vi "simple_pwm.vi"() -> ()   [LabVIEW 2017]
uses:
  lib/libbuddy/bindings/labview/utility_vi/buddy.lvlib
panel:
  out "Function Error":bool
  out "Configuration Error":bool
  out "output cluster":T1
  in  "packet":T1
  out "CH5":bool
  out "CH4":bool
  out "CH3":bool
  out "CH2":bool
  out "CH1":bool=TRUE
  out "function return":i32
  out "configure return":i32
  in  "Stream Mode":bool
  in  "PWM Mode":i32(listbox)=1
  in  "runtime":T2
  in  "CH5":u32(slide) max=65535 step=1 scale=0.0..65535.0
  in  "CH4":u32(slide) max=65535 step=1 scale=0.0..65535.0
  in  "CH3":u32(slide) max=65535 step=1 scale=0.0..65535.0
  in  "CH2":u32(slide) max=65535 step=1 scale=0.0..65535.0
  in  "CH1":u32(slide) max=65535 step=1 scale=0.0..65535.0
  in  "PWM Resolution":i32(listbox)=1
  out "PWM Sample Time":dbl
  in  "PWM Timebase":i32(listbox)=2
  out "Iterations":i32
  in  "stop":bool
  out "timing":cluster{"period":u32, "averaging":u8}
  in  "PWM Sample Rate (Hz)":dbl=10.0
  out "fw_info out":T3
  in  "timing":cluster{"period":u32, "averaging":u8}={"period"=1000000, "averaging"=0}
  in  "general":T4={"function"=2, "mode"=1, "channel_mask"=255, "resolution"=1}
  out "str_serial":string
  out "str_mfr":string
  out "str_product":string
  out "str_index_1":string
  out "handle":u64 format="%x"
  # "CONFIGURATION"
  # "DEVICE INFO"
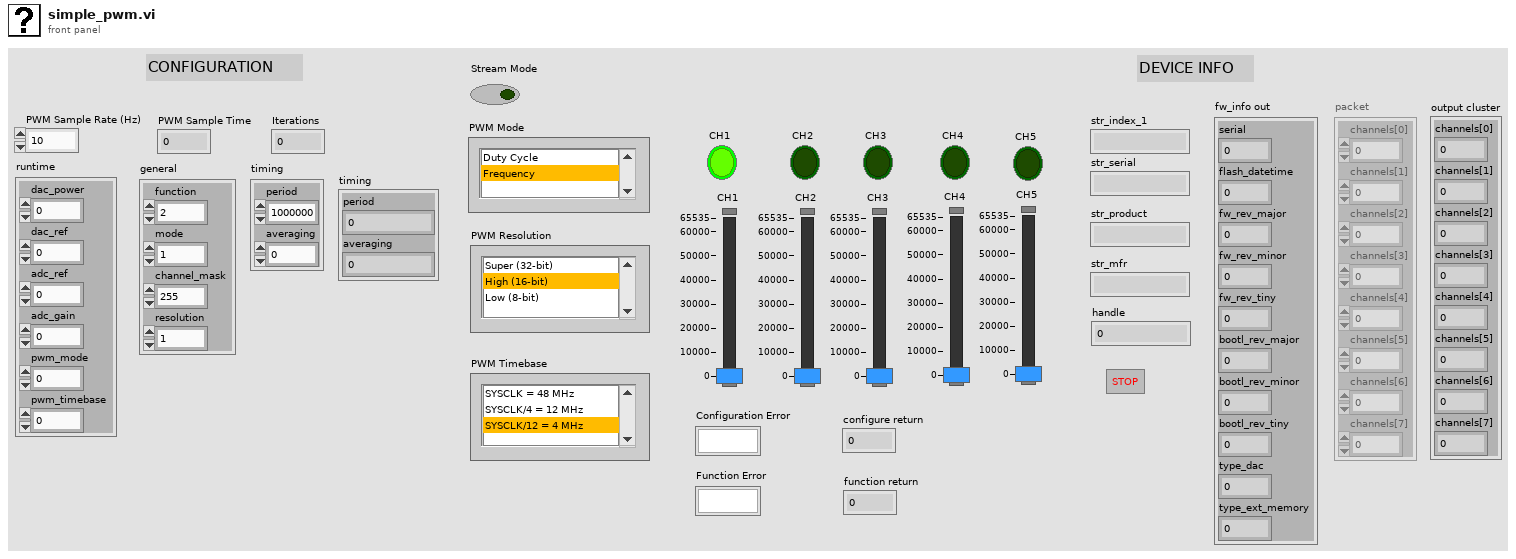
[diagram p1: front panel]
types:
  T1 = cluster{"channels[0]":u32, "channels[1]":u32, "channels[2]":u32, "channels[3]":u32, "channels[4]":u32, "channels[5]":u32, "channels[6]":u32, "channels[7]":u32}
  T2 = cluster{"dac_power":u8, "dac_ref":u8, "adc_ref":u8, "adc_gain":u8, "pwm_mode":u8, "pwm_timebase":u8}
  T3 = cluster{"serial":u32, "flash_datetime":u32, "fw_rev_major":u8, "fw_rev_minor":u8, "fw_rev_tiny":u8, "bootl_rev_major":u8, "bootl_rev_minor":u8, "bootl_rev_tiny":u8, "type_dac":u8, "type_ext_memory":u8}
  T4 = cluster{"function":u8, "mode":u8, "channel_mask":u8, "resolution":u8}
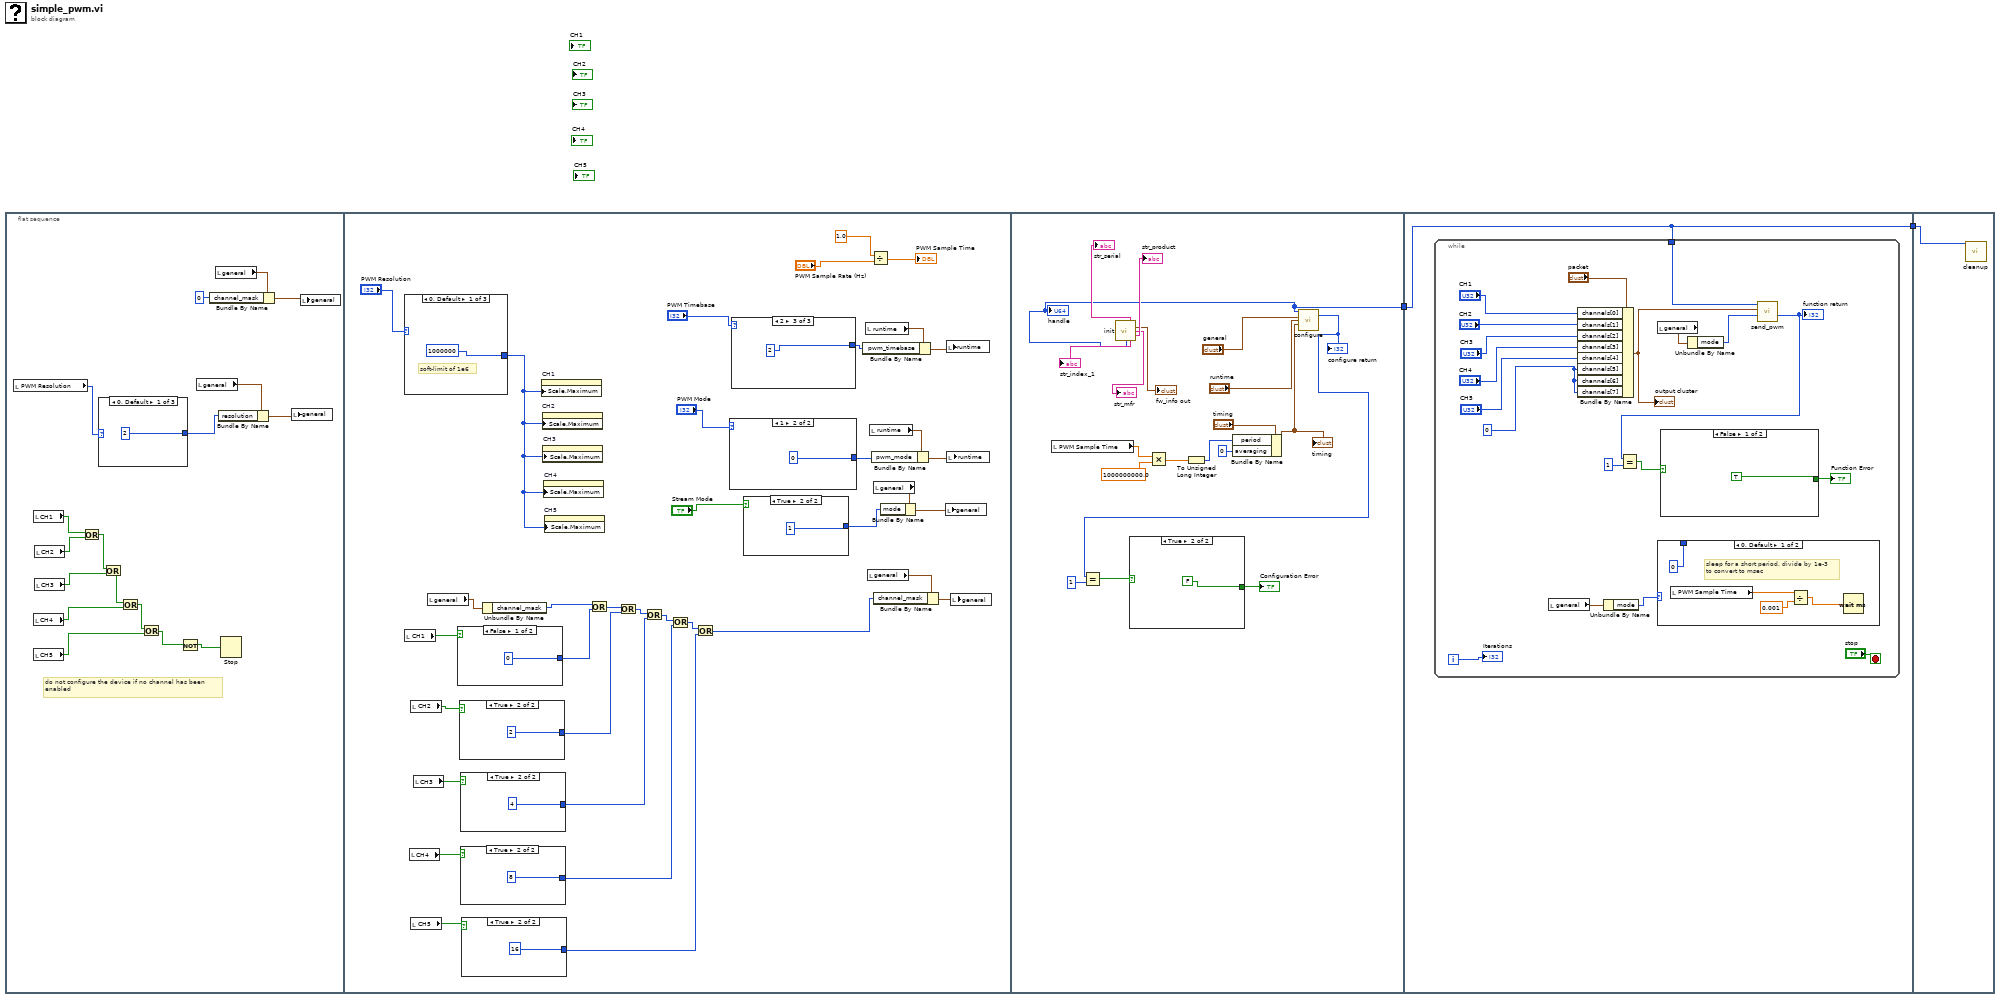
[diagram p0: block diagram]
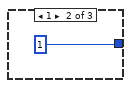
[diagram p2: hidden frame]
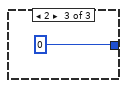
[diagram p3: hidden frame]
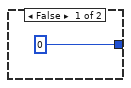
[diagram p4: hidden frame]
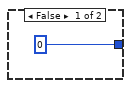
[diagram p5: hidden frame]
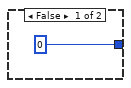
[diagram p6: hidden frame]
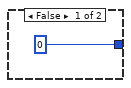
[diagram p7: hidden frame]
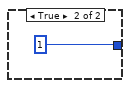
[diagram p8: hidden frame]
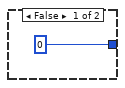
[diagram p9: hidden frame]
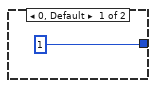
[diagram p10: hidden frame]
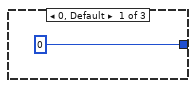
[diagram p11: hidden frame]
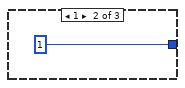
[diagram p12: hidden frame]
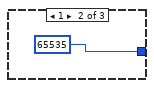
[diagram p13: hidden frame]
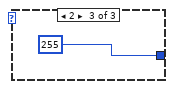
[diagram p14: hidden frame]
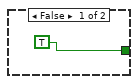
[diagram p15: hidden frame]
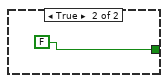
[diagram p16: hidden frame]
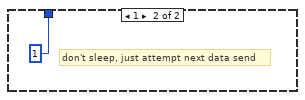
[diagram p17: hidden frame]
diagram:
  n1 = flat-sequence {
    tunnel: [w86] -> w1
    tunnel: [w100] -> w2
    tunnel: w1 -> [w100]
    tunnel: w2 -> [w127]
    frame #0 {
      # "do not configure the device if no channel has been\nenabled"
      n2 = local read "PWM Resolution"() -> (w14:i32)
      n3 = local read "CH1"() -> (w11:bool)
      n4 = local read "CH4"() -> (w7:bool)
      n5 = local read "CH5"() -> (w4:bool)
      n6 = local read "CH2"() -> (w10:bool)
      n7 = local read "CH3"() -> (w9:bool)
      n8 = Or(x=w11, y=w10) -> (x .or. y?=w8:bool)
      n9 = case shown="0, Default" w14 {
        tunnel: [u32 2 u32 1 u32 0] -> w13
        frame 0, Default {
        }
        frame 1 {
        }
        frame 2 {
        }
      }
      n10 = Or(x=w8, y=w9) -> (x .or. y?=w6:bool)
      n11 = Or(x=w6, y=w7) -> (x .or. y?=w5:bool)
      n12 = Or(x=w5, y=w4) -> (x .or. y?=w3:bool)
      n13 = Not(x=w3) -> (.not. x?=w12:bool)
      n14 = local read "general"() -> (w15:T4)
      n15 = local read "general"() -> (w18:T4)
      n16 = Bundle By Name(cluster=w18, "channel_mask"=u8 0) -> (w19:T4)
      n17 = Bundle By Name(cluster=w15, "resolution"=w13) -> (w16:T4)
      n18 = Stop(stop? (T)=w12) -> ()
      n19 = local write "general"(w16) -> ()
      n20 = local write "general"(w19) -> ()
    }
    frame #1 {
      n21 = case shown="0, Default" "PWM Resolution" {
        tunnel: [u32 1000000 u32 65535 u32 255] -> w54
        frame 0, Default {
          # "soft-limit of 1e6"
        }
        frame 1 {
        }
        frame 2 {
        }
      }
      n22 = local read "CH1"() -> (w38:bool)
      n23 = local read "CH4"() -> (w31:bool)
      n24 = local read "CH2"() -> (w35:bool)
      n25 = local read "CH5"() -> (w32:bool)
      n26 = local read "CH3"() -> (w30:bool)
      n27 = local read "general"() -> (w40:T4)
      n28 = case shown="False" w38 {
        tunnel: [u32 0 u32 1] -> w37
        frame False {
        }
        frame True {
        }
      }
      n29 = case shown="True" w35 {
        tunnel: [u32 0 u32 2] -> w34
        frame False {
        }
        frame True {
        }
      }
      n30 = case shown="True" w31 {
        tunnel: [u32 0 u32 8] -> w28
        frame False {
        }
        frame True {
        }
      }
      n31 = case shown="True" w30 {
        tunnel: [u32 0 u32 4] -> w29
        frame False {
        }
        frame True {
        }
      }
      n32 = case shown="True" w32 {
        tunnel: [u32 0 u32 16] -> w27
        frame False {
        }
        frame True {
        }
      }
      n33 = Unbundle By Name(w40) -> ("channel_mask"=w39:u8)
      n34 = property on="CH1" class="Slide (strict)"("Scale.Maximum"=w54) -> ()  [unwired: 2 in, 2 out]
      n35 = property on="CH2" class="Slide (strict)"("Scale.Maximum"=w54) -> ()  [unwired: 2 in, 2 out]
      n36 = property on="CH3" class="Slide (strict)"("Scale.Maximum"=w54) -> ()  [unwired: 2 in, 2 out]
      n37 = property on="CH4" class="Slide (strict)"("Scale.Maximum"=w54) -> ()  [unwired: 2 in, 2 out]
      n38 = property on="CH5" class="Slide (strict)"("Scale.Maximum"=w54) -> ()  [unwired: 2 in, 2 out]
      n39 = Or(x=w39, y=w37) -> (x .or. y?=w33:u32)
      n40 = Or(x=w33, y=w34) -> (x .or. y?=w26:u32)
      n41 = Or(x=w26, y=w29) -> (x .or. y?=w25:u32)
      n42 = Or(x=w25, y=w28) -> (x .or. y?=w24:u32)
      n43 = Or(x=w24, y=w27) -> (x .or. y?=w23:u32)
      n44 = case shown="1" "PWM Mode" {
        tunnel: [u32 1 u32 0] -> w47
        frame 0, Default {
        }
        frame 1 {
        }
      }
      n45 = case shown="2" "PWM Timebase" {
        tunnel: [u32 0 u32 1 u32 2] -> w52
        frame 0, Default {
        }
        frame 1 {
        }
        frame 2 {
        }
      }
      n46 = case shown="True" "Stream Mode" {
        tunnel: [u32 0 u32 1] -> w42
        frame False {
        }
        frame True {
        }
      }
      n47 = local read "runtime"() -> (w51:T2)
      n48 = Bundle By Name(cluster=w51, "pwm_timebase"=w52) -> (w50:T2)
      n49 = local read "general"() -> (w41:T4)
      n50 = local read "runtime"() -> (w49:T2)
      n51 = Divide(x=1.0, y="PWM Sample Rate (Hz)") -> (x/y=→"PWM Sample Time":dbl)
      n52 = Bundle By Name(cluster=w49, "pwm_mode"=w47) -> (w48:T2)
      n53 = local read "general"() -> (w44:T4)
      n54 = Bundle By Name(cluster=w41, "channel_mask"=w23) -> (w36:T4)
      n55 = Bundle By Name(cluster=w44, "mode"=w42) -> (w43:T4)
      n56 = local write "general"(w43) -> ()
      n57 = local write "runtime"(w50) -> ()
      n58 = local write "runtime"(w48) -> ()
      n59 = local write "general"(w36) -> ()
    }
    frame #2 {
      n60 = local read "PWM Sample Time"() -> (w84:dbl)
      n61 = call "init.vi"() -> ("str_serial"=→"str_serial":string, "fw_info out"=→"fw_info out":T3, "str_mfr"=→"str_mfr":string, "str_product"=→"str_product":string, "return type"=w86:u64, "str_index_1"=→"str_index_1":string)  [unwired: 8 in, 2 out]
      "handle" <- w86
      n62 = Multiply(x=w84, y=1000000000.0) -> (x*y=w89:dbl)
      n63 = To Unsigned Long Integer(number=w89) -> (unsigned 32bit integer=w88:u32)
      n64 = Bundle By Name(cluster="timing", "period"=w88, "averaging"=u8 0) -> (w91:cluster{"period":u32, "averaging":u8})
      "timing" <- w91
      n65 = call "configure.vi"("handle in"=w86, "general"="general", "runtime"="runtime", "timing"=w91) -> ("function return"=w82:i32)  [unwired: 7 in, 4 out]
      "configure return" <- w82
      n66 = Equal?(x=w82, y=1) -> (x = y?=w80:bool)
      n67 = case shown="True" w80 {
        tunnel: [TRUE FALSE] -> w79
        frame False {
        }
        frame True {
        }
      }
      "Configuration Error" <- w79
    }
    frame #3 {
      n68 = while {
        tunnel: w100 -> [w117]
        i -> [w118]
        stop <- "stop" stop-if-true
        w108 = u32 0
        n69 = local read "general"() -> (w116:T4)
        n70 = Bundle By Name(cluster="packet", "channels[0]"="CH1", "channels[1]"="CH2", "channels[2]"="CH3", "channels[3]"="CH4", "channels[4]"="CH5", "channels[5]"=w108, "channels[6]"=w108, "channels[7]"=w108) -> (w113:T1)
        "output cluster" <- w113
        n71 = Unbundle By Name(w116) -> ("mode"=w115:u8)
        n72 = local read "general"() -> (w106:T4)
        n73 = case shown="0, Default" w115 {
          tunnel: [u32 0 u32 1] -> _
          frame 0, Default {
            # "sleep for a short period, divide by 1e-3\nto convert to msec"
            n74 = local read "PWM Sample Time"() -> (w124:dbl)
            n75 = Divide(x=w124, y=0.001) -> (x/y=w125:dbl)
            n76 = Wait (ms)(milliseconds to wait=w125) -> ()  [unwired: 1 out]
          }
          frame 1 {
            # "don't sleep, just attempt next data send"
          }
        }
        n77 = Unbundle By Name(w106) -> ("mode"=w105:u8)
        n78 = call "send_pwm.vi"("streaming"=w105, "packet"=w113, "handle"=w117) -> ("function return"=w104:i32)  [unwired: 7 in, 1 out]
        "function return" <- w104
        n79 = Equal?(x=w104, y=1) -> (x = y?=w102:bool)
        n80 = case shown="False" w102 {
          tunnel: [TRUE FALSE] -> w101
          frame False {
          }
          frame True {
          }
        }
        "Function Error" <- w101
        "Iterations" <- w118
      }
    }
    frame #4 {
      n81 = call "cleanup.vi"("handle"=w127) -> ()  [unwired: 13 in, 2 out]
    }
  }
